vi "ULx Read (Digital 1D U16 1Chan NSamp).vi"(0 "task in":refnum<k24>, 7 "number of samples per channel":i32=-1, 9 "timeout":dbl=10.0 format="%_4g", 11 "error in":errorcluster) -> (4 "task out":refnum<k24>, 6 "data":u16[](array[numeric]), 15 "error out":errorcluster)   [LabVIEW 2020]
doc: "Reads one or more 16-bit unsigned integer samples from a task that contains a single digital input channel. Use an instance that reads 16-bit unsigned integers for devices with up to 16 lines per port."
uses:
  C:/Users/William/Documents/LV 2020 builds/LeaktestDAQ/Source-v33/ULx_LV.dll
  ULx_LV.dll
panel:
  # "sample #"
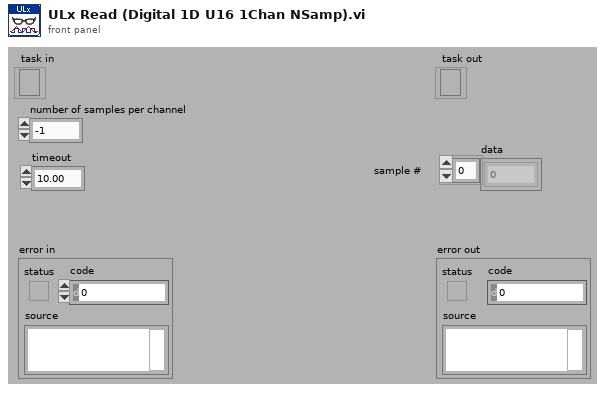
[diagram p1: front panel]
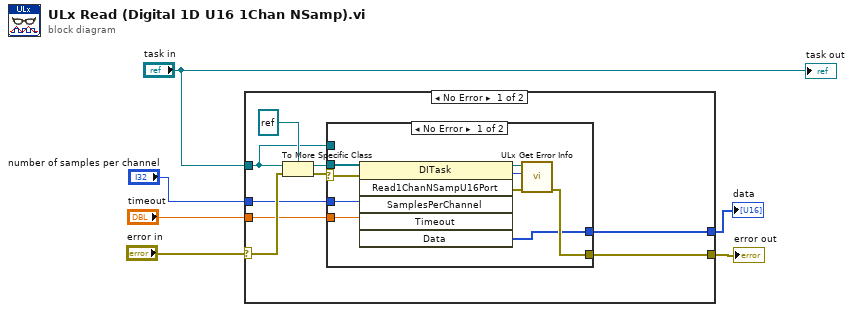
[diagram p0: block diagram]
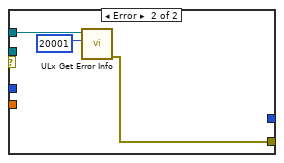
[diagram p2: hidden frame]
diagram:
  n1 = case shown="No Error" "error in" {
    selector: "error in" -> [w15 w28]
    tunnel: "task in" -> [w7 _]
    tunnel: "timeout" -> [w11 _]
    tunnel: [w10 w28] -> w4
    tunnel: "number of samples per channel" -> [w9 _]
    tunnel: [w8 _] -> w1
    frame No Error {
      n2 = To More Specific Class(target class=refnum<k24> refnum, reference=w7, error in=w15) -> (specific class reference=w12:refnum<k24>, error out=w13:errorcluster)
      n3 = case shown="No Error" w13 {
        selector: w13 -> [w23 _]
        tunnel: w12 -> [w24 _]
        tunnel: w11 -> [w19 _]
        tunnel: [w20 w25] -> w10
        tunnel: w9 -> [w18 _]
        tunnel: [w17 _] -> w8
        tunnel: w7 -> [_ w27]
        frame No Error {
          n4 = invoke class="DITask" method="Read1ChanNSampU16Port"(reference=w24, error in=w23, "SamplesPerChannel"=w18, "Timeout"=w19) -> (reference out=w21:refnum<k24>, error out=w22:errorcluster, "Read1ChanNSampU16Port"=w16:i32, "Data"=w17:u16[])  [unwired: 2 in, 2 out]
          n5 = call "ULx Get Error Info.vi"("error in"=w22, "ErrorCode"=w16, "task in"=w21) -> ("error out"=w20:errorcluster)  [unwired: 8 in]
        }
        frame Error {
          n6 = call "ULx Get Error Info.vi"("ErrorCode"=20001, "task in"=w27) -> ("error out"=w25:errorcluster)  [unwired: 9 in]
        }
      }
    }
    frame Error {
    }
  }
  "error out" <- w4
  "data" <- w1
  "task out" <- "task in"
